vi "Autonomous.vi"(11 "Call Context":T8) -> (0 "SubState 2":T3, 1 "Loop 2 Data":T2, 2 "SubState 1":T3, 3 "Loop 1 Data":T4, 5 "SubState 0":T3=enum."driver control", 7 "Loop 0 Data":T6={"State"=enum."null", "Waiting Loop"=0, "State to Wait For"=0, "Loop ID"=0, "Exit Value"=0, "X Axis"=0.0, "Y Axis"=0.0, "Z Axis"=0.0, "Mode"=enum."Arcade Drive"}, 8 "SubState 3":T1)   [LabVIEW 2014]
uses:
  typedefs/state machine/subStates.ctl
  <vilib>/Rock Robotics/WPI/DriverStation/WPI_DriverStationDerivedRobotMode.ctl
  typedefs/loop datatypes/Loop 0 Datatype.ctl
  typedefs/drive mode.ctl
  typedefs/loop datatypes/Loop 1 Datatype.ctl
  typedefs/lift/lift command.ctl
  typedefs/loop datatypes/Loop 2 Datatype.ctl
  typedefs/state machine/singleUseSubstate.ctl
  typedefs/fg_getset.ctl
  typedefs/vision/vision enable.ctl
  <vilib>/Rock Robotics/WPI/CAN/TalonSRX/WPI_CANTalonSRX_BrakeOverride.ctl
  global variables/devrefs.vi
  global variables/dashboard data.vi
panel:
  # "Autonomous Loop Data and Substates"
  # "Robot Drive"
  # "Loop 1: Lift Belts"
  # "Loop 2: Container Arm"
  # "Loop 3: Tote Pistons"
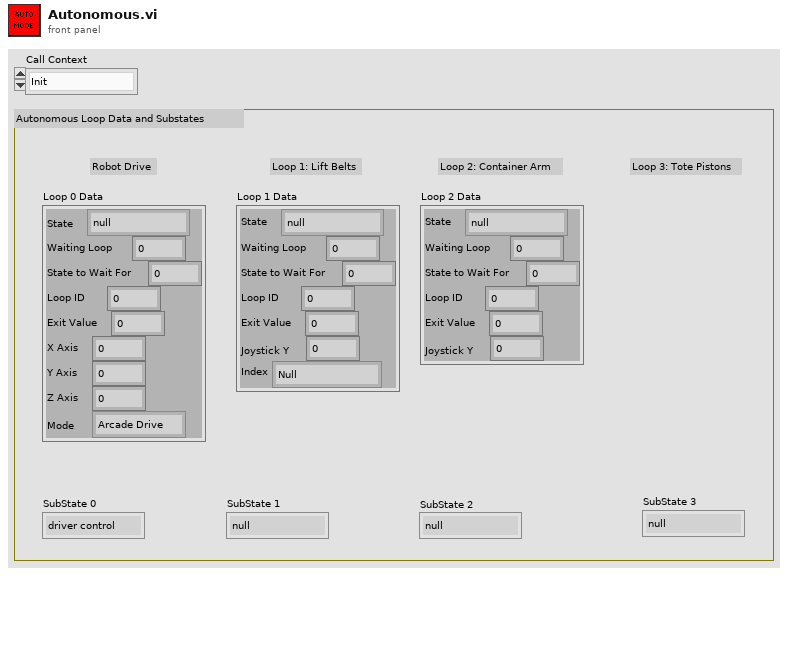
[diagram p1: front panel]
types:
  T1 = typedef "singleUseSubstate.ctl" = enum16{"null", "wait", "extend", "retract", "end"}
  T2 = typedef "Loop 2 Datatype.ctl" = cluster{"State":T3, "Waiting Loop":i32, "State to Wait For":i32, "Loop ID":i32, "Exit Value":i32, "Joystick Y":dbl}
  T3 = typedef "subStates.ctl" = enum16{"null", "wait", "driver control", "auto", "manual override", "hold position", "rotate", "test", "end"}
  T4 = typedef "Loop 1 Datatype.ctl" = cluster{"State":T3, "Waiting Loop":i32, "State to Wait For":i32, "Loop ID":i32, "Exit Value":i32, "Joystick Y":dbl, "Index":T5}
  T5 = typedef "lift command.ctl" = enum16{"Null", "Index Up", "Index Down", "Go To Home", "Pick Up Auto Stack", "Container Index Up", "Container Index Down", "Autonomous"}
  T6 = typedef "Loop 0 Datatype.ctl" = cluster{"State":T3, "Waiting Loop":i32, "State to Wait For":i32, "Loop ID":i32, "Exit Value":i32, "X Axis":dbl, "Y Axis":dbl, "Z Axis":dbl, "Mode":T7}
  T7 = typedef "drive mode.ctl" = enum16{"Left/Right X/Y Control", "Arcade Drive", "H-Drive", "H-Drive Spin", "H-Drive PID", "Autonomous"}
  T8 = typedef "WPI_DriverStationDerivedRobotMode.ctl" = enum16{"Init", "Execute", "Stop"}
  T9 = typedef "vision enable.ctl" = enum16{"Enable", "Disable", "Stop"}
  T10 = typedef "fg_getset.ctl" = enum16{"Get", "Set"}
  T11 = typedef "WPI_CANTalonSRX_BrakeOverride.ctl" = enum8{"No Override", "Override to Coast", "Override to Brake"}
  T12 = typedef "WPI_MotorControlDeviceRef.ctl" = cluster{"DeviceStatus":errorcluster, "Type":T13, "PWM":cluster{"Controller":T14, "PWM Channel":T15, "DeadBand":T16}, "CAN":cluster{"Device Number":u8, "Control Mode":T17, "Semaphore":T18, "Max Vout":dbl, "TalonSRX Control Mode":T19}, "Invert":bool, "TransformRef":T20, "InvTransformRef":T20}
  T13 = typedef "WPI_MotorControlType.ctl" = enum16{"PWM", "CAN", "CANTalonSRX"}
  T14 = typedef "FPGA_TypedefDigitalModule.ctl" = enum16{"Controller 1"}
  T15 = typedef "FPGA_DIOPWMChannel.ctl" = enum8{"PWM 0", "PWM 1", "PWM 2", "PWM 3", "PWM 4", "PWM 5", "PWM 6", "PWM 7", "PWM 8", "PWM 9", "PWM MXP 0", "PWM MXP 1", "PWM MXP 2", "PWM MXP 3", "PWM MXP 4", "PWM MXP 5", "PWM MXP 6", "PWM MXP 7", "PWM MXP 8", "PWM MXP 9", "Invalid"}
  T16 = typedef "WPI_PWMDeadband.ctl" = cluster{"Name":string, "maxPositivePwm":i32, "minPositivePwm":i32, "centerPwm":i32, "maxNegativePwm":i32, "minNegativePwm":i32, "angularRange":u16}
  T17 = typedef "WPI_CANJaguar_ControlMode.ctl" = enum8{"Percent VBus", "Current", "Speed", "Position", "Voltage"}
  T18 = typedef "Semaphore RefNum" = refnum<k1>
  T19 = typedef "WPI_CANTalonSRX_APIControlMode.ctl" = enum8{"Percent VBus", "Speed", "Position", "Slave", "Unchanged / Invalid"}
  T20 = typedef "WPI_PWMTransform_ConPane.ctl" = refnum<vi>
  T21 = typedef "WPI_GyroDevRef.ctl" = cluster{"DevStatus":errorcluster, "Analog Module":T22, "Analog Channel":T23, "Offset":dbl, "Gain (VoltsPerDegree/Second)":dbl}
  T22 = typedef "FPGA_TypedefAnalogModule.ctl" = enum16{"Controller 1"}
  T23 = typedef "FPGA_AIChannel.ctl" = enum8{"AI 0", "AI 1", "AI 2", "AI 3", "AI MXP 0", "AI MXP 1", "AI MXP 2", "AI MXP 3", "Invalid"}
  T24 = enum32{"None", "Autonomous 1 (Drive)", "Autonomous 2 (3 Tote)", "Autonomous 3 (Container)"}
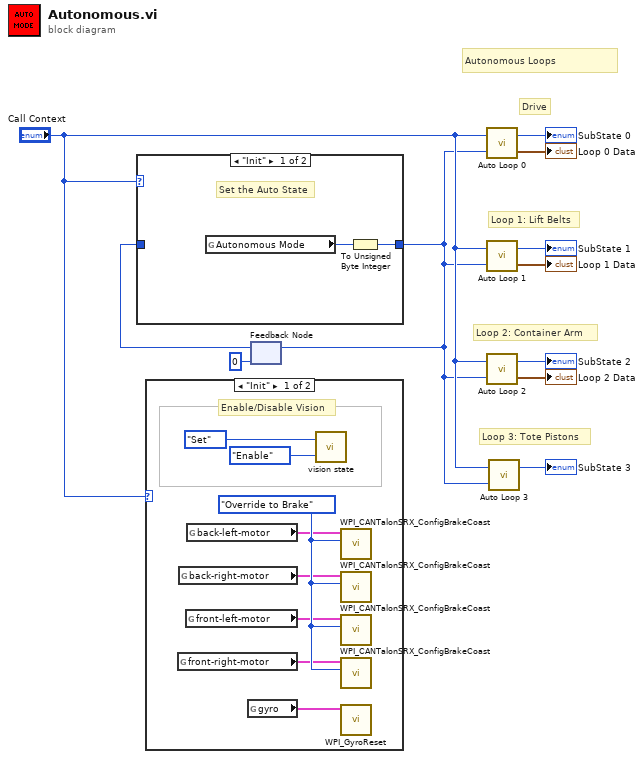
[diagram p0: block diagram]
diagram:
  # "Loop 3: Tote Pistons"
  # "Autonomous Loops"
  # "Loop 2: Container Arm"
  # "Loop 1: Lift Belts"
  # "Drive"
  n1 = case shown="\"Init\"" "Call Context" {
    frame "Init" {
      w17 = WPI_CANTalonSRX_BrakeOverride."Override to Brake" ("Brake / Coast Mode")
      # "Enable/Disable Vision"
      n2 = global read "devrefs.vi" "front-right-motor"() -> (w13:T12)
      n3 = global read "devrefs.vi" "back-right-motor"() -> (w15:T12)
      n4 = global read "devrefs.vi" "front-left-motor"() -> (w14:T12)
      n5 = global read "devrefs.vi" "back-left-motor"() -> (w16:T12)
      n6 = global read "devrefs.vi" "gyro"() -> (w12:T21)
      n7 = call "vision state.vi"("State In"=vision_enable."Enable" ("Action"), "Menu"=fg_getset."Set") -> ()  [unwired: 2 out]
      n8 = call <vilib>:"WPI_CANTalonSRX_ConfigBrakeCoast.vi"("Brake / Coast Mode"=w17, "CAN Talon SRX Ref"=w16) -> ()  [unwired: 8 in, 2 out]
      n9 = call <vilib>:"WPI_CANTalonSRX_ConfigBrakeCoast.vi"("Brake / Coast Mode"=w17, "CAN Talon SRX Ref"=w15) -> ()  [unwired: 8 in, 2 out]
      n10 = call <vilib>:"WPI_CANTalonSRX_ConfigBrakeCoast.vi"("Brake / Coast Mode"=w17, "CAN Talon SRX Ref"=w14) -> ()  [unwired: 8 in, 2 out]
      n11 = call <vilib>:"WPI_CANTalonSRX_ConfigBrakeCoast.vi"("Brake / Coast Mode"=w17, "CAN Talon SRX Ref"=w13) -> ()  [unwired: 8 in, 2 out]
      n12 = call <vilib>:"WPI_GyroReset.vi"("GyroDevRef"=w12) -> ()  [unwired: 9 in, 2 out]
    }
    frame "Execute", Default {
    }
  }
  n13 = feedback #1(u8 0 ("Read Auto State")) -> (w4:u8)
  n14 = case shown="\"Init\"" "Call Context" {
    tunnel: [w20 w22] -> w1
    tunnel: w4 -> [_ w22]
    frame "Init" {
      # "Set the Auto State"
      n15 = global read "dashboard data.vi" "Autonomous Mode"() -> (w21:T24)
      n16 = To Unsigned Byte Integer(number=w21) -> (unsigned 8bit integer=w20:u8)
    }
    frame "Execute", Default {
    }
  }
  n17 = feedback-in #1(w1) -> ()
  n18 = call "Auto Loop 0.vi"("Auto State"=w1, "Call Context"="Call Context") -> ("Loop 0 Data"=→"Loop 0 Data":T6, "SubState 0"=→"SubState 0":T3)
  n19 = call "Auto Loop 1.vi"("Auto State"=w1, "Call Context"="Call Context") -> ("Loop 1 Data"=→"Loop 1 Data":T4, "SubState 1"=→"SubState 1":T3)
  n20 = call "Auto Loop 2.vi"("Auto State"=w1, "Call Context"="Call Context") -> ("Loop 2 Data"=→"Loop 2 Data":T2, "SubState 2"=→"SubState 2":T3)
  n21 = call "Auto Loop 3.vi"("Auto State"=w1, "Call Context"="Call Context") -> ("SubState 3"=→"SubState 3":T1)  [unwired: 1 in]
